vi "ROI grp-Case-Save ROI groups table to file.vi"(8 "error in (no error)":errorcluster) -> (0 "error out":errorcluster)   [LabVIEW 2020]
uses:
  Experiment header interface/Typedefs/Save-Load-Save as-Load last enum.ctl
  Globals/gl_ROI grp window globals.vi
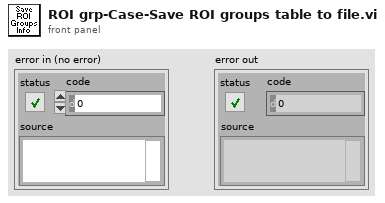
[diagram p1: front panel]
types:
  T1 = typedef "Save-Load-Save as-Load last enum.ctl" = enum16{"Save file", "Save file as", "Load file", "Load last file"}
  T2 = typedef "ROI grp-window ctrl refs.ctl" = cluster{"This VI":refnum<vi>, "Pane":refnum<vi>, "Table":refnum<vi>}
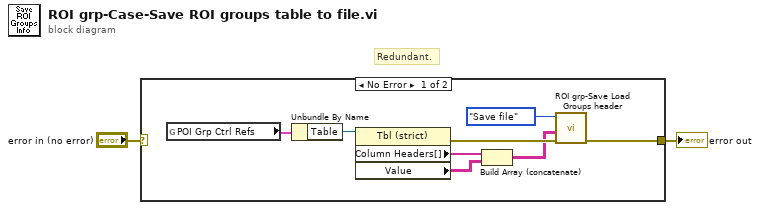
[diagram p0: block diagram]
diagram:
  # "Redundant."
  n1 = case shown="No Error" "error in (no error)" {
    selector: "error in (no error)" -> [_ w11]
    tunnel: [w3 w11] -> w1
    frame No Error {
      n2 = global read "gl_ROI grp window globals.vi" "POI Grp Ctrl Refs"() -> (w4:T2)
      n3 = Unbundle By Name(w4) -> ("Table"=w10:refnum<vi>)
      n4 = property on="Property Node" class="Tbl (strict)"(reference=w10) -> (error out=w7:errorcluster, "Column Headers[]"=w9:string[], "Value"=w8:string[][])  [unwired: 1 in, 1 out]
      n5 = Build Array (concatenate)(w9, w8) -> (w6:string[][])
      n6 = call "ROI grp-Save Load Groups header.vi"("error in (no error)"=w7, "POI groups header file data (in)"=w6, "Function"=Save-Load-Save_as-Load_last_enum."Save file") -> ("error out"=w3:errorcluster)  [unwired: 6 in, 2 out]
    }
    frame Error {
    }
  }
  "error out" <- w1
